vi "Aula_1_24022026.vi"() -> ()   [LabVIEW 2024]
panel:
  in  "Boolean":bool
  out "Numeric":i32
  out "x*y":dbl
  out "°C":dbl(slide) scale=0.0..100.0
  in  "°F":dbl(slide) scale=0.0..110.0
  in  "stop":bool
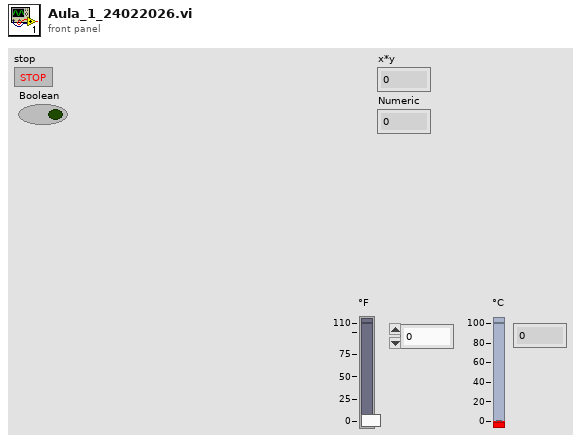
[diagram p1: front panel]
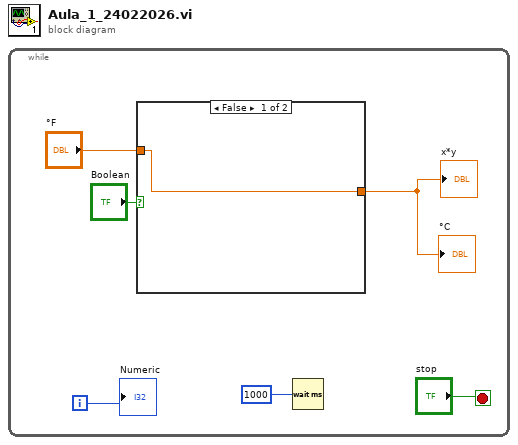
[diagram p0: block diagram]
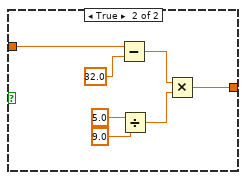
[diagram p2: hidden frame]
diagram:
  n1 = while {
    i -> [w5]
    stop <- "stop" stop-if-true
    n2 = case shown="False" "Boolean" {
      tunnel: [w7 w9] -> w4
      tunnel: "°F" -> [w7 w8]
      frame False {
      }
      frame True {
        n3 = Subtract(x=w8, y=32.0) -> (x-y=w11:dbl)
        n4 = Divide(x=5.0, y=9.0) -> (x/y=w10:dbl)
        n5 = Multiply(x=w11, y=w10) -> (x*y=w9:dbl)
      }
    }
    "x*y" <- w4
    "°C" <- w4
    n6 = Wait (ms)(milliseconds to wait=u32 1000) -> ()  [unwired: 1 out]
    "Numeric" <- w5
  }
